vi "Number To String.vi"(1 "Digits":i32, 2 "Number":T1={"Array Num"=[1, 2, 3], "Decimal Index"=0, "stop"=FALSE}) -> (0 "String":string)   [LabVIEW 2025]
uses:
  Number.ctl
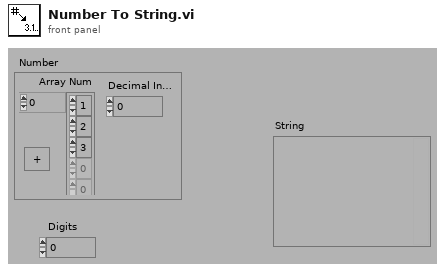
[diagram p1: front panel]
types:
  T1 = typedef "Number.ctl" = cluster{"Array Num":i8[], "Decimal Index":i32, "stop":bool}
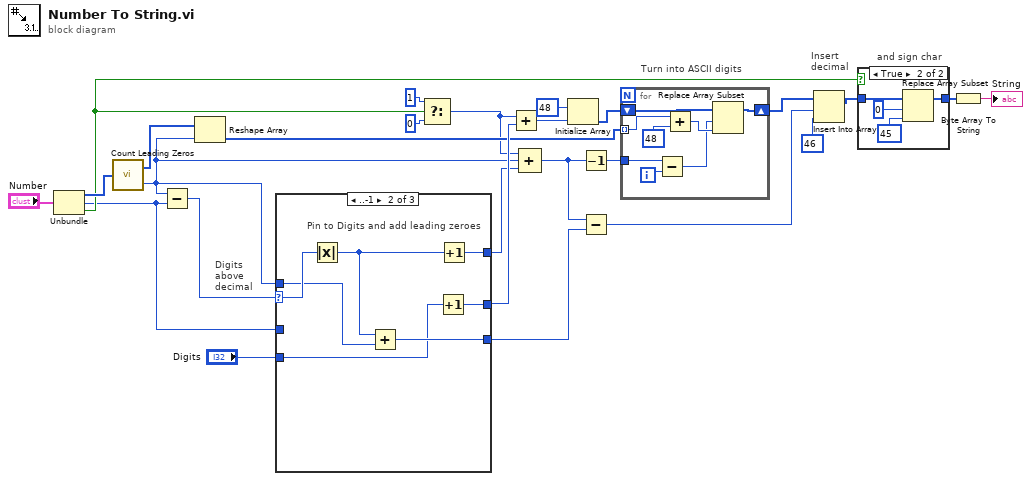
[diagram p0: block diagram]
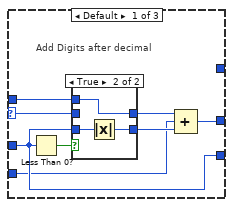
[diagram p2: hidden frame]
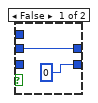
[diagram p3: hidden frame]
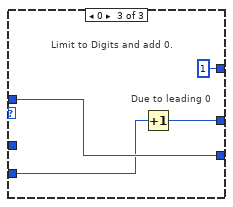
[diagram p4: hidden frame]
diagram:
  # "Turn into ASCII digits"
  # "Insert\ndecimal"
  # "and sign char"
  # "Digits\nabove\ndecimal"
  n1 = Unbundle("Number") -> ("Array Num"=w22:i8[], "Decimal Index"=w12:i32, "stop"=w17:bool)
  n2 = call "Count Leading Zeros.vi"("Array Num"=w22) -> ("Array Dup"=w15:i8[], "NonZero Count"=w1:i32)
  n3 = Subtract(x=w1, y=w12) -> (x-y=w14:i32)
  n4 = Reshape Array(w15, w1) -> (w18:i8[])
  n5 = case shown="..-1" w14 {
    selector: w14 -> [w28 w44 _]
    tunnel: "Digits" -> [w30 w40 w47]
    tunnel: [w32 w46 w49] -> w26
    tunnel: w1 -> [w29 w41 w48]
    tunnel: w12 -> [w33 _ _]
    tunnel: [w33 w43 w48] -> w3
    tunnel: [_ w45 1 ("x")] -> w2
    frame Default {
      # "Add Digits after decimal"
      n6 = Less Than 0?(x=w33) -> (x < 0?=w34:bool)
      n7 = case shown="True" w34 {
        tunnel: w33 -> [_ w39]
        tunnel: [0 w38] -> w31
        tunnel: w29 -> [_ w37]
        tunnel: w28 -> [w35 _]
        tunnel: [w35 w37] -> w27
        frame False {
        }
        frame True {
          n8 = Absolute Value(x=w39) -> (abs(x)=w38:i32)
        }
      }
      n9 = Compound Arithmetic op=ADD(w27, w30, w31) -> (w32:i32)
    }
    frame ..-1 {
      # "Pin to Digits and add leading zeroes"
      n10 = Absolute Value(x=w44) -> (abs(x)=w42:i32)
      n11 = Add(x=w42, y=w41) -> (x+y=w43:i32)
      n12 = Increment(x=w40) -> (x+1=w46:i32)
      n13 = Increment(x=w42) -> (x+1=w45:i32)
    }
    frame 0 {
      # "Due to leading 0"
      # "Limit to Digits and add 0."
      n14 = Increment(x=w47) -> (x+1=w49:i32)
    }
  }
  n15 = Select(t=1, s=w17, f=0) -> (s? t:f=w10:i32)
  n16 = Add(x=w10, y=w26) -> (x+y=w11:i32)
  n17 = Compound Arithmetic op=ADD(w10, w1, w2) -> (w5:i32)
  n18 = Initialize Array(u8 48, w11) -> (w16:u8[])
  n19 = Decrement(x=w5) -> (x-1=w9:i32)
  n20 = Subtract(x=w5, y=w3) -> (x-y=w4:i32)
  n21 = for {
    shift-right: [w54] -> w7
    shift-left: w16 -> [w58]
    tunnel: w18 -> [w56] mode=indexing
    tunnel: w9 -> [w53]
    i -> [w51]
    n22 = Subtract(x=w53, y=w51) -> (x-y=w52:i32)
    n23 = Add(x=w56, y=i8 48) -> (x+y=w57:i8)
    n24 = Replace Array Subset(array=w58, new element=w57, index=w52) -> (w54:u8[])
  }
  n25 = Insert Into Array(array=w7, index=w4, new element=i8 46) -> (w6:u8[])
  n26 = case shown="True" w17 {
    tunnel: [w59 w61] -> w19
    tunnel: w6 -> [w59 w62]
    frame False {
    }
    frame True {
      n27 = Replace Array Subset(array=w62, new element=i8 45, index=u8 0) -> (w61:u8[])
    }
  }
  n28 = Byte Array To String(unsigned byte array=w19) -> (string=→"String":string)
